vi "save_profile.vi"(7 "Motor Adress":T1(ring)=enum."3", 8 "error in (no error)":errorcluster, 10 "Profile Data":i32[](array[numeric]), 11 "VISA ressource in":refnum<visa-resource-name>="COM1") -> (0 "error out":errorcluster={"status"=FALSE, "code"=1073676294, "source"="VISA Read in write_read.vi"}, 3 "VISA ressource out":refnum<visa-resource-name>)   [LabVIEW 2013]
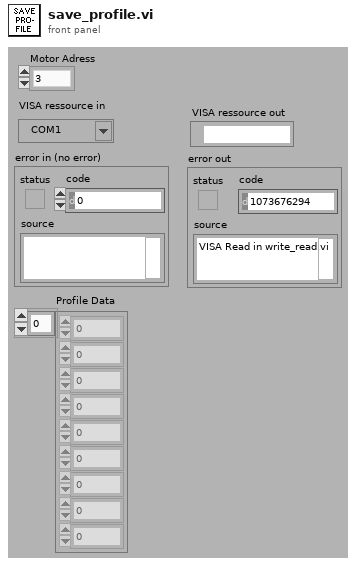
[diagram p1: front panel]
types:
  T1 = enum16{"All", "1", "2", "3", "4", "5", "6", "7", "8"}
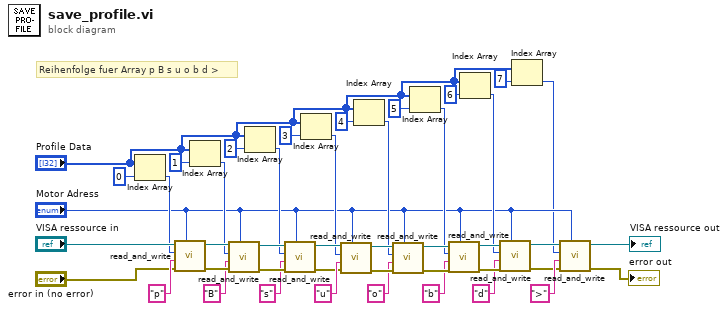
[diagram p0: block diagram]
diagram:
  # "Reihenfolge fuer Array p B s u o b d >"
  n1 = Index Array(array="Profile Data", index=0) -> (element=w23:i32)
  n2 = call "read_and_write.vi"("Motor Adress"="Motor Adress", "error in (no error)"="error in (no error)", "Command"="p" ("string"), "value"=w23, "VISA ressource in"="VISA ressource in") -> ("error out"=w43:errorcluster, "VISA ressource out"=w44:refnum<visa-resource-name>)  [unwired: 3 in, 2 out]
  n3 = Index Array(array="Profile Data", index=1) -> (element=w22:i32)
  n4 = call "read_and_write.vi"("Motor Adress"="Motor Adress", "error in (no error)"=w43, "Command"="B" ("command letter"), "value"=w22, "VISA ressource in"=w44) -> ("error out"=w41:errorcluster, "VISA ressource out"=w42:refnum<visa-resource-name>)  [unwired: 3 in, 2 out]
  n5 = Index Array(array="Profile Data", index=2) -> (element=w21:i32)
  n6 = call "read_and_write.vi"("Motor Adress"="Motor Adress", "error in (no error)"=w41, "Command"="s" ("string"), "value"=w21, "VISA ressource in"=w42) -> ("error out"=w27:errorcluster, "VISA ressource out"=w26:refnum<visa-resource-name>)  [unwired: 3 in, 2 out]
  n7 = Index Array(array="Profile Data", index=3) -> (element=w20:i32)
  n8 = call "read_and_write.vi"("Motor Adress"="Motor Adress", "error in (no error)"=w27, "Command"="u" ("command letter"), "value"=w20, "VISA ressource in"=w26) -> ("error out"=w39:errorcluster, "VISA ressource out"=w40:refnum<visa-resource-name>)  [unwired: 3 in, 2 out]
  n9 = Index Array(array="Profile Data", index=4) -> (element=w19:i32)
  n10 = call "read_and_write.vi"("Motor Adress"="Motor Adress", "error in (no error)"=w39, "Command"="o" ("command letter"), "value"=w19, "VISA ressource in"=w40) -> ("error out"=w38:errorcluster, "VISA ressource out"=w37:refnum<visa-resource-name>)  [unwired: 3 in, 2 out]
  n11 = Index Array(array="Profile Data", index=5) -> (element=w10:i32)
  n12 = call "read_and_write.vi"("Motor Adress"="Motor Adress", "error in (no error)"=w38, "Command"="b" ("command letter"), "value"=w10, "VISA ressource in"=w37) -> ("error out"=w36:errorcluster, "VISA ressource out"=w35:refnum<visa-resource-name>)  [unwired: 3 in, 2 out]
  n13 = Index Array(array="Profile Data", index=6) -> (element=w18:i32)
  n14 = call "read_and_write.vi"("Motor Adress"="Motor Adress", "error in (no error)"=w36, "Command"="d", "value"=w18, "VISA ressource in"=w35) -> ("error out"=w8:errorcluster, "VISA ressource out"=w6:refnum<visa-resource-name>)  [unwired: 3 in, 2 out]
  n15 = Index Array(array="Profile Data", index=7) -> (element=w1:i32)
  n16 = call "read_and_write.vi"("Motor Adress"="Motor Adress", "error in (no error)"=w8, "Command"=">", "value"=w1, "VISA ressource in"=w6) -> ("error out"=→"error out":errorcluster, "VISA ressource out"=→"VISA ressource out":refnum<visa-resource-name>)  [unwired: 3 in, 2 out]
